vi "PH_4_Pos_Selector.calc Position.vi"(0 "i ref in":refnum<vi>, 5 "error in (no error)":errorcluster) -> (14 "i ref out":refnum<vi>, 19 "error out":errorcluster)   [LabVIEW 2014, in "PH_4_Pos_Selector.lvlib"]
doc: "This VI calculates the current position and writes it to own attributes, if it has changed."
uses:
  PH_4_Pos_Selector.lvlib
  PH_4_Pos_Selector.Position Selector.ctl
  lib.lib/DimLVEvent/LVDimInterface/LVDimInterface.lvlib
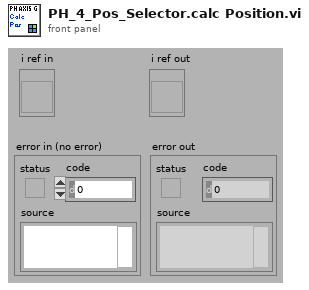
[diagram p1: front panel]
types:
  T1 = typedef "PH_4_Pos_Selector.lvlib/PH_4_Pos_Selector.Position.ctl" = cluster{"Axis 1":dbl, "Axis 2":dbl}
  T2 = typedef "PH_4_Pos_Selector.lvlib/PH_4_Pos_Selector.i attribute.ctl" = cluster{"GUI Refs":cluster{"Position I":refnum<vi>, "Position II":refnum<vi>, "Position III":refnum<vi>, "Position IV":refnum<vi>, "rel. Mode?":refnum<vi>, "Define Selector":refnum<vi>}, "Current Position":T3, "Service ID Position":i32, "Position Array":T1[], "Description Array":string[], "relative Mode":bool, "Wanted Define Selector Position":string}
  T3 = typedef "PH_4_Pos_Selector.lvlib/PH_4_Pos_Selector.Position Selector.ctl" = u16
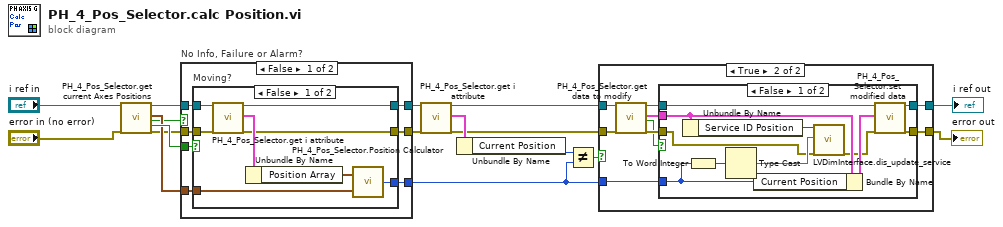
[diagram p0: block diagram]
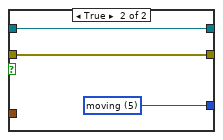
[diagram p2: hidden frame]
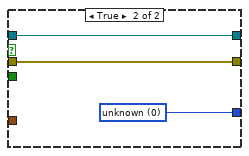
[diagram p3: hidden frame]
diagram:
  n1 = call "PH_4_Pos_Selector.get current Axes Positions.vi"("VI in"="i ref in", "error in (no error)"="error in (no error)") -> ("VI out"=w9:refnum<vi>, "Current Axes Positions"=w10:T1, "No Info, Failure oder Alarm?"=w1:bool, "Moving?"=w13:bool, "error out"=w8:errorcluster)  [unwired: 13 in]
  n2 = case "No Info, Failure or Alarm?" shown="False" w1 {
    tunnel: [w24 w38] -> w15
    tunnel: w13 -> [w23 _]
    tunnel: w10 -> [w22 _]
    tunnel: w9 -> [w21 w37]
    tunnel: w8 -> [w20 w36]
    tunnel: [w19 w37] -> w4
    tunnel: [w18 w36] -> w2
    frame False {
      n3 = case "Moving?" shown="False" w23 {
        tunnel: w22 -> [w25 _]
        tunnel: [w32 w33] -> w24
        tunnel: w21 -> [w30 w35]
        tunnel: w20 -> [w29 w34]
        tunnel: [w28 w35] -> w19
        tunnel: [w27 w34] -> w18
        frame False {
          n4 = call "PH_4_Pos_Selector.get i attribute.vi"("i ref in"=w30, "error in (no error)"=w29) -> ("i ref out"=w28:refnum<vi>, "i attribute"=w31:T2, "error out"=w27:errorcluster)  [unwired: 15 in]
          n5 = Unbundle By Name(w31) -> ("Position Array"=w26:T1[])
          n6 = call "PH_4_Pos_Selector.Position Calculator.vi"("Current Axes Positions"=w25, "Position Array"=w26) -> ("Current Position"=w32:T3)
        }
        frame True {
          w33 = T3 5 items=["unknown", "Position I", "Position II", "Position III", "Position IV", "moving"] ("Current Position")
        }
      }
    }
    frame True {
      w38 = T3 0 items=["unknown", "Position I", "Position II", "Position III", "Position IV", "moving"] ("Current Position")
    }
  }
  n7 = call "PH_4_Pos_Selector.get i attribute.vi"("i ref in"=w4, "error in (no error)"=w2) -> ("i ref out"=w5:refnum<vi>, "i attribute"=w7:T2, "error out"=w3:errorcluster)  [unwired: 15 in]
  n8 = Unbundle By Name(w7) -> ("Current Position"=w6:T3)
  n9 = Not Equal?(x=w6, y=w15) -> (x != y?=w14:bool)
  n10 = case shown="True" w14 {
    tunnel: w3 -> [w39 w49]
    tunnel: [w39 w47] -> w17
    tunnel: [w40 w46] -> w16
    tunnel: w5 -> [w40 w45]
    tunnel: w15 -> [_ w41]
    frame False {
    }
    frame True {
      n11 = call "PH_4_Pos_Selector.get data to modify.vi"("i ref in"=w45, "error in (no error)"=w49) -> ("i ref out"=w44:refnum<vi>, "i attribute"=w43:T2, "timed out"=w42:bool, "error out"=w48:errorcluster)  [unwired: 14 in]
      n12 = case shown="False" w42 {
        tunnel: w48 -> [w50 w61]
        tunnel: [w60 w61] -> w47
        tunnel: [w59 w62] -> w46
        tunnel: w44 -> [w58 w62]
        tunnel: w43 -> [w56 _]
        tunnel: w41 -> [w52 _]
        frame False {
          n13 = Unbundle By Name(w56) -> ("Service ID Position"=w55:i32)
          n14 = To Word Integer(number=w52) -> (16bit integer=w51:i16)
          n15 = Type Cast(x=w51) -> (*(type *) &x=w53:string)  [unwired: 1 in]
          n16 = Bundle By Name(cluster=w56, "Current Position"=w52) -> (w57:T2)
          n17 = call "LVDimInterface.dis_update_service.vi"("my_serviceID"=w55, "data"=w53, "error in (no error)"=w50) -> ("error out"=w54:errorcluster)  [unwired: 14 in, 2 out]
          n18 = call "PH_4_Pos_Selector.set modified data.vi"("i ref in"=w58, "i attribute"=w57, "error in (no error)"=w54) -> ("i ref out"=w59:refnum<vi>, "error out"=w60:errorcluster)  [unwired: 15 in]
        }
        frame True {
        }
      }
    }
  }
  "error out" <- w17
  "i ref out" <- w16
